vi "Cross Spectrum No Averaging (Mag-Phase).vi"(0 "scaled signal X [EUx]":waveform(dbl), 1 "scaled signal Y [EUy]":waveform(dbl), 2 "window":T3=1 items=["None"=0, "Hanning"=1, "Hamming"=2, "Blackman-Harris"=3, "Exact Blackman"=4, "Blackman"=5, "Flat Top"=6, "4 Term B-Harris "=7, "7 Term B-Harris"=8, "Low Sidelobe"=9, "Force - Exponential"=10, "Blackman Nuttall"=11, "Triangle"=30, "Bartlett-Hanning"=31, "Bohman"=32, "Parzen"=33, "Welch"=34, "Kaiser"=60, "Dolph-Chebyshev"=61, "Gaussian"=62], 4 "view":T2={"dB On (T)"=TRUE, "unwrap phase (F)"=FALSE, "convert to degree (T)"=TRUE}, 5 "error in (no error)":errorcluster, 8 "force/exp settings":T1={"force window [%]"=50.0, "exp window [%]"=10.0} {"exp window [%]" min=0.0 max=100.0 format="%.2f"; "force window [%]" min=0.0 max=100.0 format="%.2f"}) -> (16 "phase [degrees]":cluster{"f0":dbl, "df":dbl, "phase":sgl[]} {"phase" format="%.2f"; "df" format="%.2f"; "f0" format="%.2f"}, 17 "phase unit label":string, 19 "error out":errorcluster)   [LabVIEW 2017, in "VibrationAnalysisFunctions.lvlib"]
doc: "Computes the cross power spectrum of <B>scaled signal X [EUx]</B> and <B>scaled signal Y [EUy]</B>. Results are returned in magnitude and phase."
uses:
  <vilib>/addons/InsightCM/Utilities/Analysis/Vibration/VibrationAnalysisFunctions.lvlib
  <vilib>/addons/_NISVFA/_Shared subVIs/Controls/svc_Window [Dual FFT].ctl
  <vilib>/addons/_NISVFA/_Shared subVIs/Controls/svc_Spectrum Info.ctl
  <vilib>/addons/_NISVFA/_Shared subVIs/Controls/svc_X-Axis Units.ctl
  <vilib>/addons/_NISVFA/_Shared subVIs/Controls/svc_Spectrum Type.ctl
  <vilib>/addons/_NISVFA/_Shared subVIs/Controls/svc_Engineering Units Text Ring.ctl
  <vilib>/addons/_NISVFA/_Shared subVIs/Controls/svc_Weighting Filter Text Ring.ctl
  <vilib>/addons/_NISVFA/_Shared subVIs/Controls/svc_Complimentary Spectrum Units.ctl
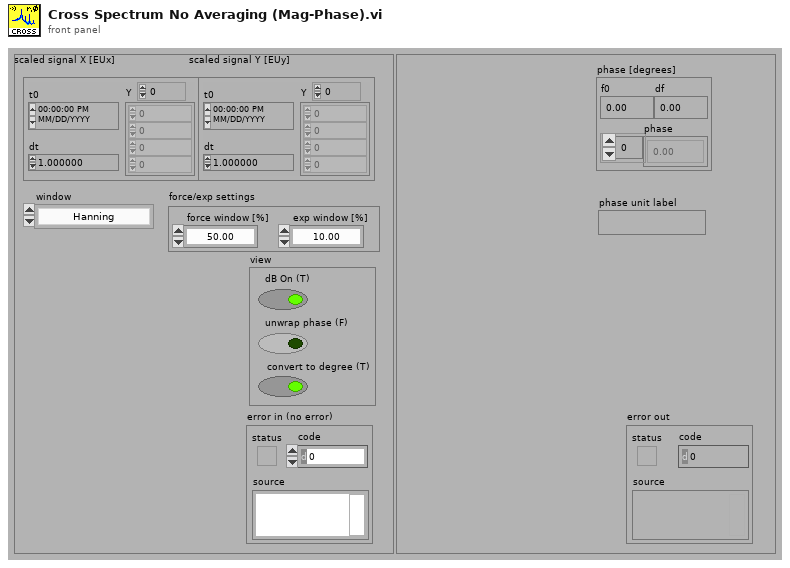
[diagram p1: front panel]
types:
  T1 = cluster{"force window [%]":dbl, "exp window [%]":dbl}
  T2 = cluster{"dB On (T)":bool, "unwrap phase (F)":bool, "convert to degree (T)":bool}
  T3 = typedef "svc_Window [Dual FFT].ctl" = u32
  T4 = typedef "svc_Spectrum Info.ctl" = cluster{"channel name":string, "description":string, "x-axis units":T5, "spectral info":cluster{"spectrum type":T6, "linear/dB":enum16{"linear", "dB"}, "window":u16, "window size":i32, "FFT size":i32}, "engineering units":T7, "custom label":string, "dB reference [EU]":dbl, "peak units":enum16{"rms", "peak", "peak-peak"}, "weighting filter":T8, "spectral density?":bool, "unit label":string, "spectrum skewed?":bool, "complimentary spectrum units":T9}
  T5 = typedef "svc_X-Axis Units.ctl" = u16
  T6 = typedef "svc_Spectrum Type.ctl" = enum16{"FFT Spectrum [complex]", "Amplitude [Magnitude]", "Power [Magnitude^2]", "Cross Spectrum [complex]", "Frequency Response [Complex]"}
  T7 = typedef "svc_Engineering Units Text Ring.ctl" = u16
  T8 = typedef "svc_Weighting Filter Text Ring.ctl" = u16
  T9 = typedef "svc_Complimentary Spectrum Units.ctl" = enum16{"none", "radians", "degrees", "cycles", "imaginary"}
  T10 = cluster{"f0":dbl, "df":dbl, "complex spectrum":cdb[]}
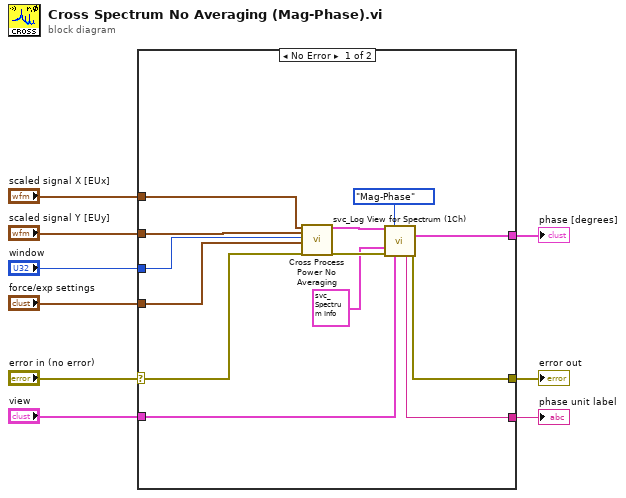
[diagram p0: block diagram]
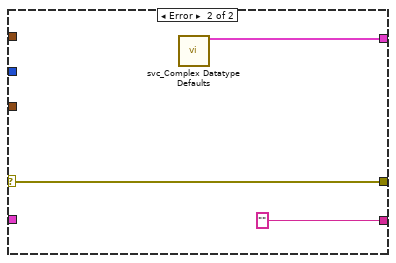
[diagram p2: hidden frame]
diagram:
  n1 = case shown="No Error" "error in (no error)" {
    selector: "error in (no error)" -> [w15 w25]
    tunnel: "window" -> [w13 _]
    tunnel: "view" -> [w22 _]
    tunnel: [w16 w25] -> w7
    tunnel: [w20 w23] -> w6
    tunnel: "force/exp settings" -> [w14 _]
    tunnel: "scaled signal X [EUx]" -> [w11 _]
    tunnel: "scaled signal Y [EUy]" -> [w12 _]
    tunnel: [w21 "" ("Unit label [Mag - Real]")] -> w1
    frame No Error {
      n2 = call <vilib>:"Cross Process Power No Averaging.vi"("input signal X"=w11, "input signal Y"=w12, "window"=w13, "force/exp settings"=w14, "error in (no error)"=w15) -> ("complex spectrum"=w19:T10, "error out"=w18:errorcluster)  [unwired: 13 in]
      n3 = call <vilib>:"svc_Log View for Spectrum (1Ch).vi"("complex spectrum"=w19, "View"=enum16{"Mag-Phase", "Real-Imaginary"}."Mag-Phase", "spectrum info in"=T4 {"channel name"="", "description"="", "x-axis units"=0, "spectral info"={"spectrum type"=enum."Power [Magnitude^2]", "linear/dB"=enum."linear", "window"=0, "window size"=0, "FFT size"=0}, "engineering units"=1, "custom label"="", "dB reference [EU]"=0.0, "peak units"=enum."rms", "weighting filter"=0, "spectral density?"=FALSE, "unit label"="", "spectrum skewed?"=FALSE, "complimentary spectrum units"=enum."none"}, "error in (no error)"=w18, "view"=w22) -> ("phase or imag"=w20:cluster{"f0":dbl, "df":dbl, dbl[]}, "unit label [phase or imag]"=w21:string, "error out"=w16:errorcluster)  [unwired: 5 in, 3 out]
    }
    frame Error {
      n4 = call <vilib>:"svc_Complex Datatype Defaults.vi"() -> ("empty spectrum"=w23:cluster{"f0":dbl, "df":dbl, "magnitude":dbl[]})  [unwired: 11 in, 8 out]
    }
  }
  "error out" <- w7
  "phase [degrees]" <- w6
  "phase unit label" <- w1
